vi "Server Main.vi"   [LabVIEW 2020, in "Chat Server.lvclass"]
uses:
  Chat Server.lvclass
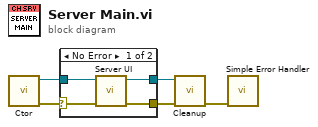
[diagram p0: block diagram]
diagram:
  n1 = call "Ctor.vi"() -> ("error out"=w5:errorcluster, "Chat Server out"=w4:refnum<class "Chat Server.lvclass">)  [unwired: 10 in]
  n2 = case shown="No Error" w5 {
    selector: w5 -> [w8 w10]
    tunnel: w4 -> [w9 w11]
    tunnel: [w7 w11] -> w2
    tunnel: [w6 w10] -> w3
    frame No Error {
      n3 = call "Server UI.vi"("error in (no error)"=w8, "Chat Server in"=w9) -> ("error out"=w6:errorcluster, "Chat Server out"=w7:refnum<class "Chat Server.lvclass">)  [unwired: 8 in]
    }
    frame Error {
    }
  }
  n4 = call "Cleanup.vi"("error in (no error)"=w3, "Chat Server in"=w2) -> ("error out"=w1:errorcluster)  [unwired: 8 in, 1 out]
  n5 = call <vilib>:"Simple Error Handler.vi"("error in (no error)"=w1) -> ()  [unwired: 4 in, 5 out]
